vi "uTTA_Calibration_ISense.vi"(5 "CommandQueue":refnum<queue>, 6 "error in":errorcluster, 7 "AR488_in":refnum<visa-resource-name>, 8 "DataQueue":refnum<queue>, 9 "TDMS_FileIn":refnum<k34>) -> (0 "error out":errorcluster, 1 "AR488_out":refnum<visa-resource-name>, 2 "Abort":bool, 3 "TDMS_FileOut":refnum<k34>)   [LabVIEW 2021]
uses:
  <vilib>/Utility/miscctls.llb/LVPointTypeDef.ctl
  <vilib>/Analysis/6fits.llb/Curve Fitting Criteria.ctl
  19661e02-a619-439f-9162-2f55fd6be45e.vi
  <vilib>/Analysis/NI_AALPro.lvlib
panel:
  in  "Abort":bool
  out "ISEN Cal.":cluster{"Ref_Voltage":dbl, "mean":dbl}(graph)
  out "ISEN DAC Offset":dbl format="%#_6pA"
  out "ISEN DAC Residue":dbl caption="Residue" format="%.3p"
  out "ISEN DAC slope":dbl format="%#_4pA/Digit"
  in  "VerifyEachCh":bool caption="Verify for each channel"
  in  "Start DAC ISEN":bool
  in  "ISEN DAC Inc":i32=1000 caption="DAC Incements" min=0 max=32767 step=1 format="%d Counts/Step"
  out "Status":string="Exit"
  # "1. Connect the DMM in current measurement mode between the positive terminal of JP101.x and Ground \n2. Connect a ground lead to the outer Conductor of the BNC line to provide propper grounding\n3. Start the calibration"
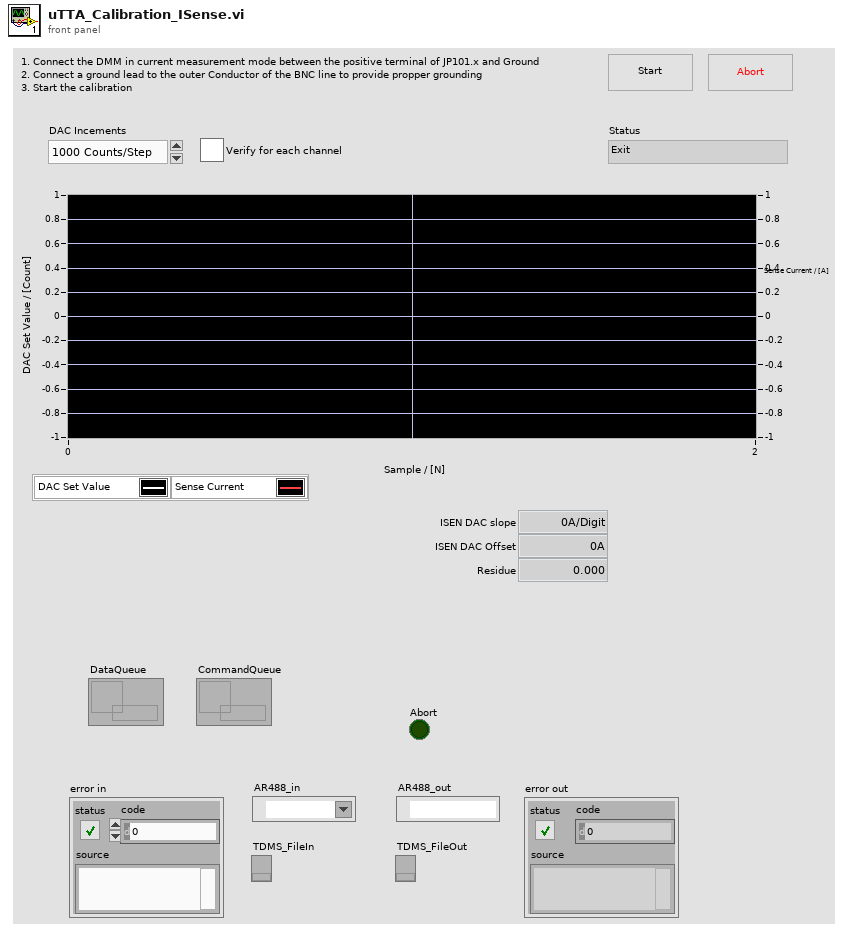
[diagram p1: front panel]
types:
  T1 = typedef "LVPointTypeDef.ctl" = cluster{"Horizontal":i16, "Vertical":i16}
  T2 = typedef "NI_AALPro.lvlib/Curve Fitting Criteria.ctl" = u16
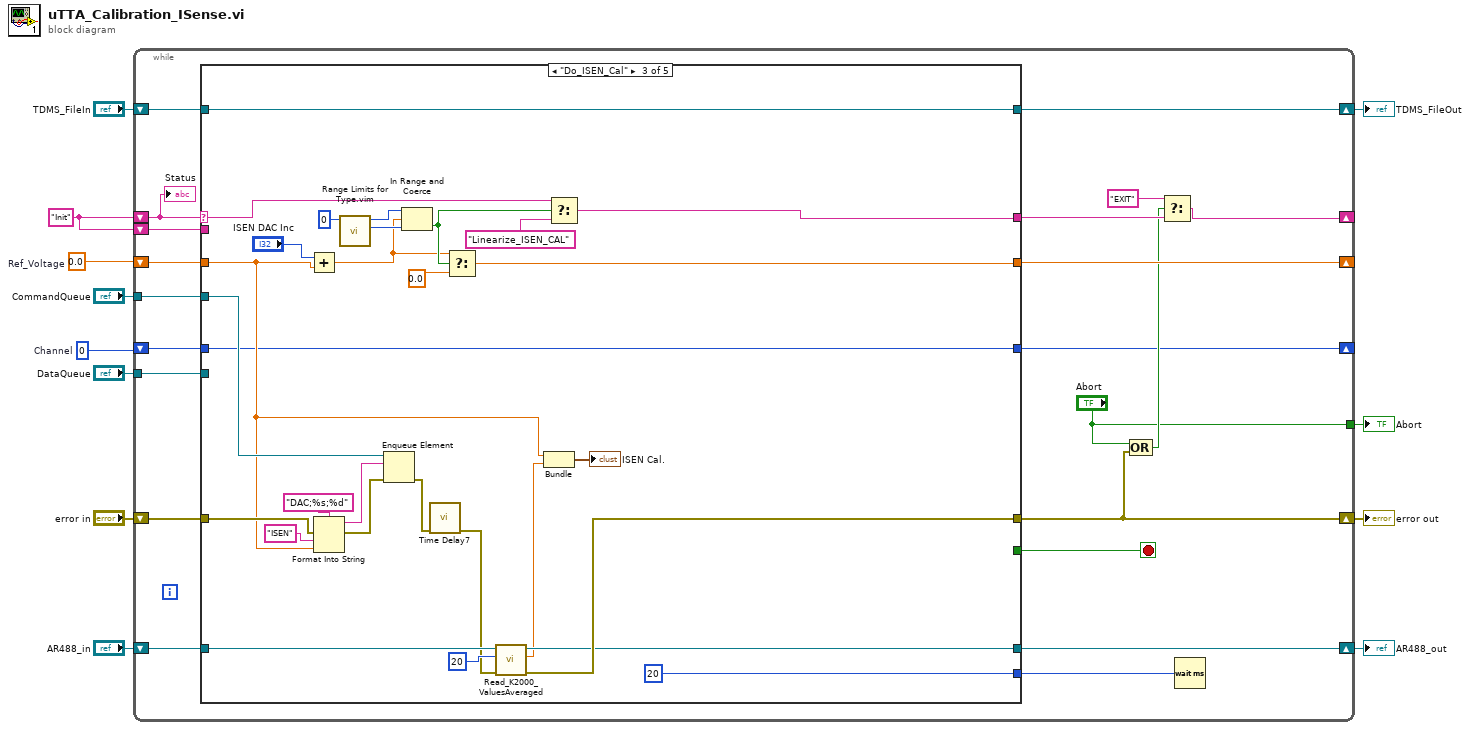
[diagram p0: block diagram]
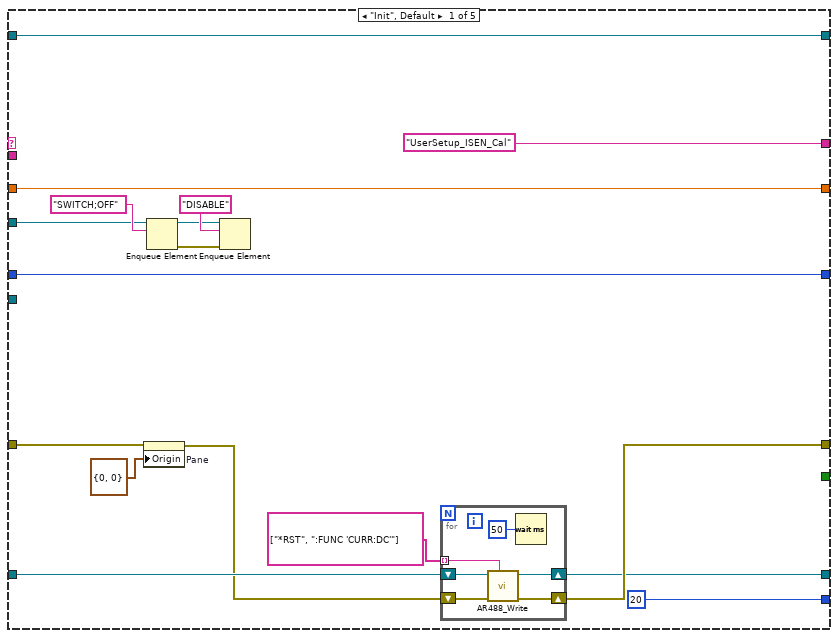
[diagram p2: hidden frame]
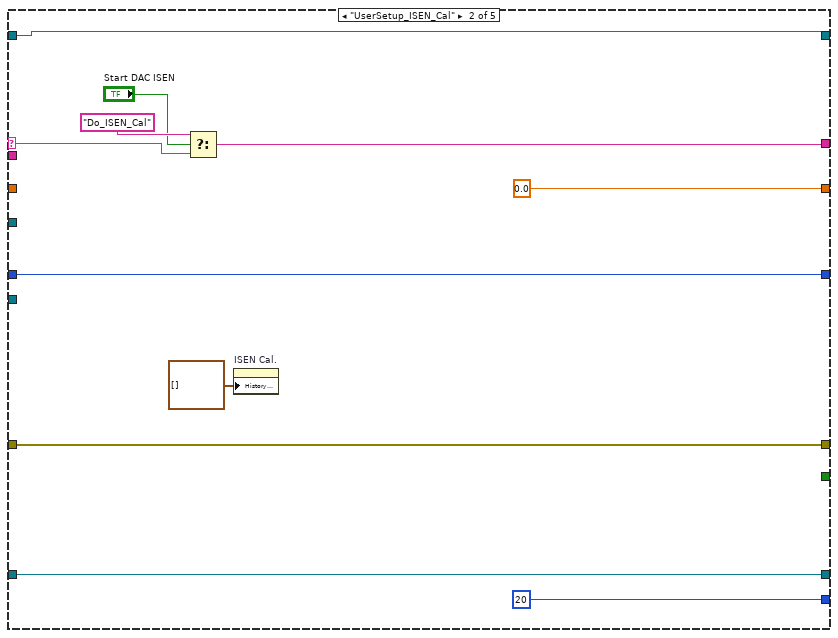
[diagram p3: hidden frame]
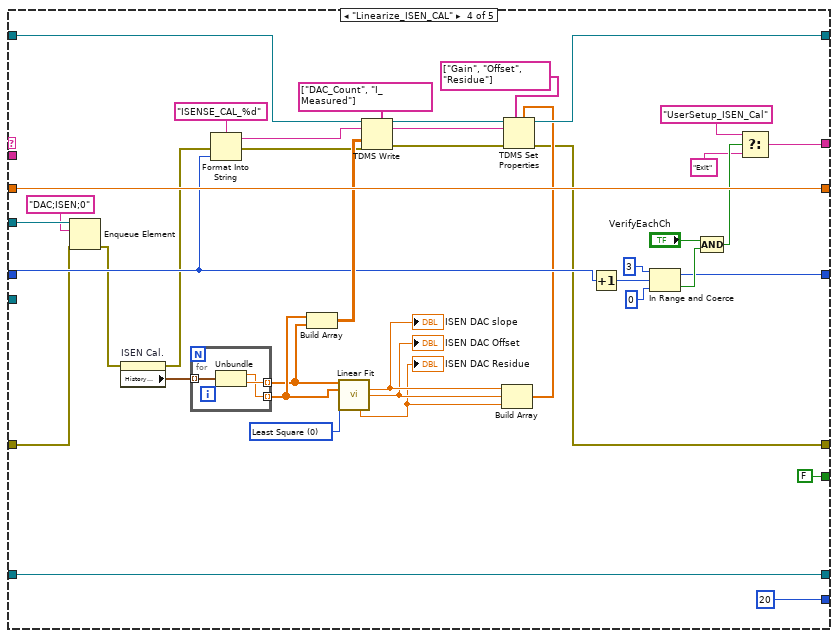
[diagram p4: hidden frame]
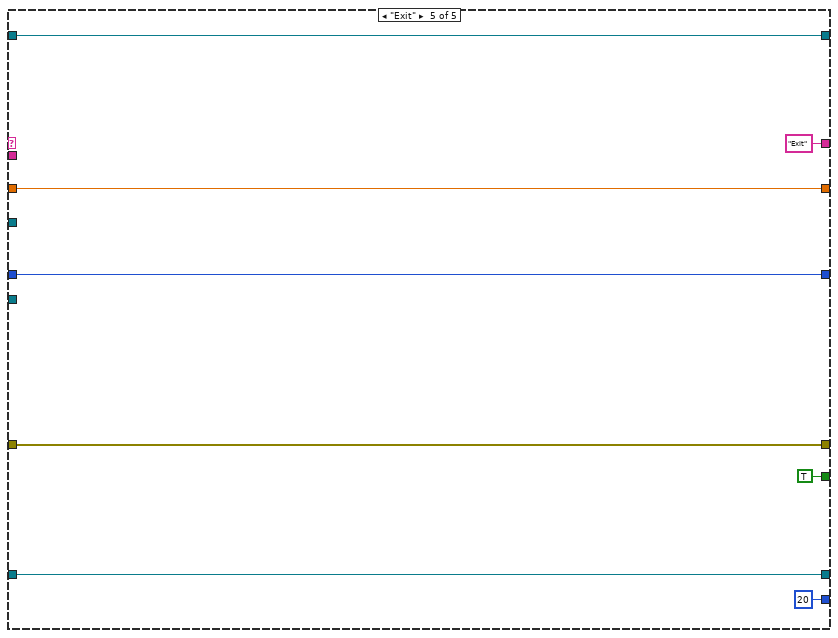
[diagram p5: hidden frame]
diagram:
  w10 = 0  # Channel
  w12 = 0.0  # Ref_Voltage
  w11 = "Init"
  n1 = while {
    shift-right: [w22] -> _
    shift-left: w11 -> [w31]
    shift-right: [w14] -> w9
    shift-left: "error in" -> [w33]
    shift-right: [w30] -> w3
    shift-left: "AR488_in" -> [w29]
    shift-left: w11 -> [w28]
    tunnel: "CommandQueue" -> [w27]
    tunnel: "DataQueue" -> [w26]
    shift-right: [w24] -> _
    shift-left: w12 -> [w25]
    shift-right: [w18] -> w5
    shift-left: "TDMS_FileIn" -> [w17]
    shift-right: [w15] -> _
    shift-left: w10 -> [w16]
    tunnel: ["Abort"] -> w1
    stop <- w19 stop-if-true
    n2 = case shown="\"Do_ISEN_Cal\"" w31 {
      selector: w31 -> [_ w61 w72 _ _]
      tunnel: [_ _ _ FALSE TRUE] -> w19
      tunnel: w33 -> [w39 w58 w91 w99 w147]
      tunnel: ["UserSetup_ISEN_Cal" ("t") w60 w78 w126 "Exit" ("f")] -> w23
      tunnel: [w46 w58 w81 w102 w147] -> w14
      tunnel: [u32 20 u32 20 u32 20 u32 20 u32 20] -> w32
      tunnel: [w45 w67 w80 w136 w146] -> w30
      tunnel: w29 -> [w43 w67 w79 w136 w146]
      tunnel: w28 -> [_ _ _ _ _]
      tunnel: w27 -> [w34 _ w95 w101 _]
      tunnel: w26 -> [_ _ _ _ _]
      tunnel: w25 -> [w49 _ w77 w135 w145]
      tunnel: [w49 0.0 w85 w135 w145] -> w24
      tunnel: [w42 w63 w96 w115 w144] -> w18
      tunnel: w17 -> [w42 w63 w96 w114 w144]
      tunnel: w16 -> [w44 w62 w73 w108 w143]
      tunnel: [w44 w62 w73 w127 w143] -> w15
      frame "Init", Default {
        n3 = property on="Pane" class="Pane"(error in=w39, "Origin"=T1 {"Horizontal"=0, "Vertical"=0}) -> (error out=w40:errorcluster)  [unwired: 1 in, 1 out]
        n4 = Enqueue Element(queue=w34, element="SWITCH;OFF") -> (queue out=w36:refnum<queue>, error out=w35:errorcluster)  [unwired: 2 in, 1 out]
        n5 = Enqueue Element(queue=w36, element="DISABLE", error in (no error)=w35) -> ()  [unwired: 1 in, 3 out]
        n6 = for {
          tunnel: string[] ["*RST", ":FUNC 'CURR:DC'"] -> [w55] mode=indexing
          shift-right: [w53] -> w45
          shift-left: w43 -> [w56]
          shift-right: [w52] -> w46
          shift-left: w40 -> [w54]
          n7 = call "AR488_Write.vi"("write"=w55, "error in (no error)"=w54, "VISA Refnum in"=w56) -> ("error out"=w52:errorcluster, "VISA Refnum out"=w53:refnum<visa-resource-name>)  [unwired: 7 in]
          n8 = Wait (ms)(milliseconds to wait=u32 50) -> ()  [unwired: 1 out]
        }
      }
      frame "UserSetup_ISEN_Cal" {
        n9 = Select(t="Do_ISEN_Cal", s="Start DAC ISEN", f=w61) -> (s? t:f=w60:string)
        n10 = property on="ISEN Cal." class="WFChart (strict)"("History Data"=cluster{"Ref_Voltage":dbl, "mean":dbl}[] []) -> ()  [unwired: 2 in, 2 out]
      }
      frame "Do_ISEN_Cal" {
        n11 = Add(x="ISEN DAC Inc", y=w77) -> (x+y=w71:dbl)
        n12 = Format Into String(format string="DAC;%s;%d" ("element"), error in=w91, "ISEN" ("input 1"), w77) -> (resulting string=w93:string, error out=w90:errorcluster)  [unwired: 1 in]
        n13 = call "Range Limits for Type.vim"("type"=u16 0) -> ("minimum value for type"=w87:u16, "maximum value for type"=w86:u16)  [unwired: 9 in]
        n14 = Enqueue Element(queue=w95, element=w93, error in (no error)=w90) -> (error out=w69:errorcluster)  [unwired: 1 in, 2 out]
        n15 = In Range and Coerce(upper limit=w86, x=w71, lower limit=w87) -> (In Range?=w84:bool)  [unwired: 1 out]
        n16 = call "Time Delay7"("error in (no error)"=w69) -> ("error out"=w68:errorcluster)  [unwired: 10 in]
        n17 = Select(t=w71, s=w84, f=0.0 ("t")) -> (s? t:f=w85:dbl)
        n18 = call "Read_K2000_ValuesAveraged.vi"("error in"=w68, "No. Averaged Values"=20, "VISA Refnum in"=w79) -> ("error out"=w81:errorcluster, "mean"=w76:dbl, "VISA Refnum out"=w80:refnum<visa-resource-name>)  [unwired: 6 in]
        n19 = Bundle("Ref_Voltage"=w77, "mean"=w76) -> (→"ISEN Cal.":cluster{"Ref_Voltage":dbl, "mean":dbl})  [unwired: 1 in]
        n20 = Select(t=w72, s=w84, f="Linearize_ISEN_CAL" ("t")) -> (s? t:f=w78:string)
      }
      frame "Linearize_ISEN_CAL" {
        w120 = T2 0 items=["Least Square", "Least Absolute Residual", "Bisquare"] ("method")
        n21 = Enqueue Element(queue=w101, element="DAC;ISEN;0", error in (no error)=w99) -> (error out=w100:errorcluster)  [unwired: 1 in, 2 out]
        n22 = property on="ISEN Cal." class="WFChart (strict)"(error in=w100) -> (error out=w103:errorcluster, "History Data"=w119:cluster{"Ref_Voltage":dbl, "mean":dbl}[])  [unwired: 1 in, 1 out]
        n23 = for {
          tunnel: w119 -> [w139] mode=indexing
          tunnel: [w138] -> w112 mode=indexing
          tunnel: [w137] -> w113 mode=indexing
          n24 = Unbundle(w139) -> ("Ref_Voltage"=w137:dbl, "mean"=w138:dbl)
        }
        n25 = Format Into String(format string="ISENSE_CAL_%d", error in=w103, w108) -> (resulting string=w107:string, error out=w104:errorcluster)  [unwired: 1 in]
        n26 = Build Array(w113, w112) -> (w111:dbl[][])
        n27 = call <vilib>:"Linear Fit.vi"("Y"=w112, "X"=w113, "method"=w120) -> ("slope"=w123:dbl, "intercept"=w122:dbl, "residue"=w121:dbl)  [unwired: 8 in, 2 out]
        "ISEN DAC Offset" <- w122
        "ISEN DAC Residue" <- w121
        "ISEN DAC slope" <- w123
        n28 = TDMS Write(0:w114, 5:w107, 7:string[] ["DAC_Count", "I_Measured"], 9:w111, 11:w104) -> (4:w118:refnum<k34>, 6:w106:string, 15:w117:errorcluster)  [unwired: 1 in, 1 out]
        n29 = Build Array(w123, w122, w121) -> (w105:dbl[])
        n30 = TDMS Set Properties(5:w105, 7:string[] ["Gain", "Offset", "Residue"] ("property names"), 8:w117, 10:w106, 11:w118) -> (0:w102:errorcluster, 3:w115:refnum<k34>)  [unwired: 1 in, 2 out]
        n31 = Increment(x=w108) -> (x+1=w128:i32)
        n32 = In Range and Coerce(upper limit=3, x=w128, lower limit=0) -> (coerced(x)=w127:i32, In Range?=w134:bool)
        n33 = Compound Arithmetic op=AND("VerifyEachCh", w134) -> (w133:bool)
        n34 = Select(t="UserSetup_ISEN_Cal", s=w133, f="Exit") -> (s? t:f=w126:string)
      }
      frame "Exit" {
      }
    }
    n35 = Compound Arithmetic op=OR("Abort", w14) -> (w20:bool)
    n36 = Select(t="EXIT", s=w20, f=w23) -> (s? t:f=w22:string)
    n37 = Wait (ms)(milliseconds to wait=w32) -> ()  [unwired: 1 out]
    "Status" <- w31
  }
  "error out" <- w9
  "TDMS_FileOut" <- w5
  "AR488_out" <- w3
  "Abort" <- w1
